vi "Configure Measurement.vi"(7 "range (-1.0: Auto)":dbl=-1.0 format="%^.2e", 8 "error in (no error)":errorcluster, 9 "absolute resolution (0.001)":dbl=0.001 format="%^.2e", 10 "measurement function (DC Volts)":i32(ring)=1 items=["DC Volts"=1, "AC Volts"=2, "DC Current"=3, "AC Current"=4, "2 Wire Resistance"=5, "4 Wire Resistance"=101, "AC + DC Volts"=106, "AC + DC Current"=107, "Frequency"=104, "Period"=105, "Temperature"=108], 11 "IVI_DMM in":refnum<class "IVI_DMM.lvclass">) -> (0 "error out":errorcluster, 3 "IVI_DMM out":refnum<class "IVI_DMM.lvclass">)   [LabVIEW 2013, in "IVI_DMM.lvlib" / "IVI_DMM.lvclass"]
doc: "This VI configures the common properties of the DMM. These properties include the measurement function, maximum range, and resolution."
uses:
  IVI_DMM.lvclass
  IVI_DMM.lvclass/IVI_DMM.ctl
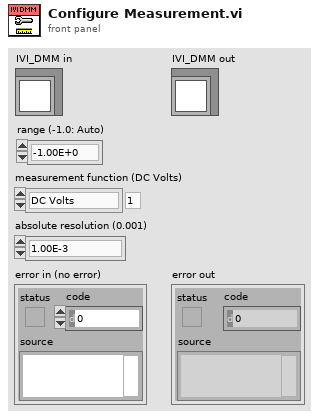
[diagram p1: front panel]
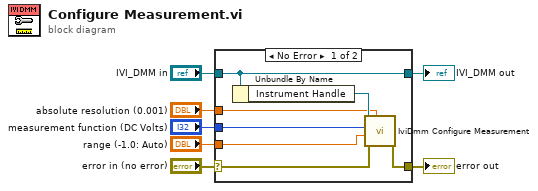
[diagram p0: block diagram]
diagram:
  n1 = case shown="No Error" "error in (no error)" {
    selector: "error in (no error)" -> [w9 w16]
    tunnel: [w8 w16] -> w6
    tunnel: [w14 w15] -> w4
    tunnel: "IVI_DMM in" -> [w14 w15]
    tunnel: "absolute resolution (0.001)" -> [w12 _]
    tunnel: "measurement function (DC Volts)" -> [w11 _]
    tunnel: "range (-1.0: Auto)" -> [w10 _]
    frame No Error {
      n2 = Unbundle By Name(w14) -> ("Instrument Handle"=w13:refnum<k15>)
      n3 = call <vilib>:"IviDmm Configure Measurement.vi"("absolute resolution (0.001)"=w12, "error in (no error)"=w9, "range (-1.0: Auto)"=w10, "measurement function (DC Volts)"=w11, "instrument handle"=w13) -> ("error out"=w8:errorcluster)  [unwired: 5 in, 1 out]
    }
    frame Error {
    }
  }
  "error out" <- w6
  "IVI_DMM out" <- w4
